vi "sv_UFF58 Check Channel Names.vi"(0 "abscissa channel name":string, 5 "ordinate numerator channel name":string, 7 "ordinate denominator channel name":string) -> (4 "abscissa channel name out":string, 6 "ordinate numerator channel name out":string, 8 "ordinate denominator channel name out":string)   [LabVIEW 2017, in "SoundVib_UFF58.lvlib"]
uses:
  <vilib>/addons/Sound and Vibration/svt_UFF58/SoundVib_UFF58.lvlib
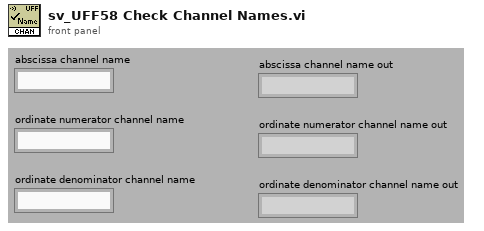
[diagram p1: front panel]
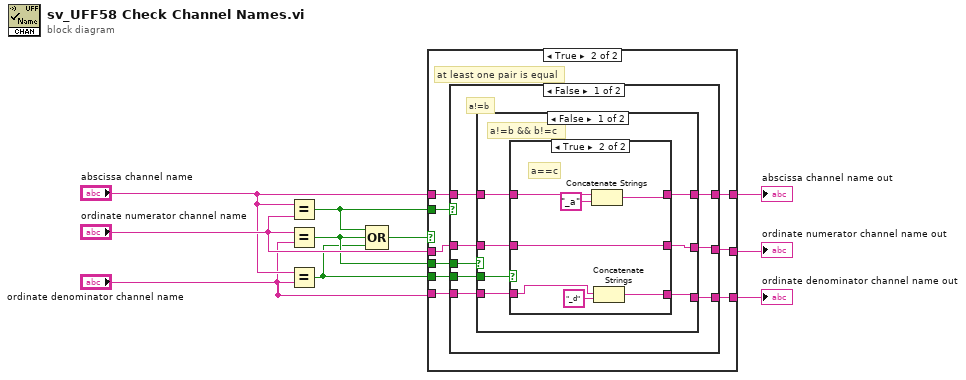
[diagram p0: block diagram]
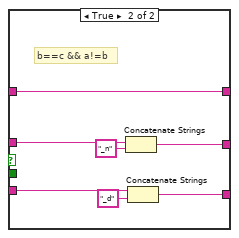
[diagram p4: hidden frame]
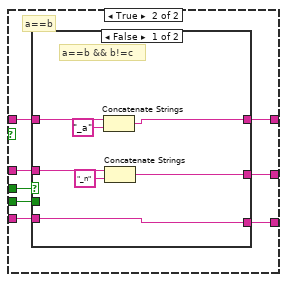
[diagram p5: hidden frame]
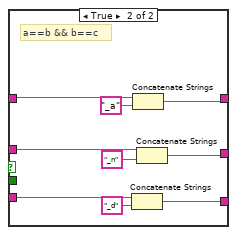
[diagram p6: hidden frame]
diagram:
  n1 = Equal?(x="abscissa channel name", y="ordinate numerator channel name") -> (x = y?=w6:bool)
  n2 = Equal?(x="ordinate numerator channel name", y="ordinate denominator channel name") -> (x = y?=w5:bool)
  n3 = Equal?(x="abscissa channel name", y="ordinate denominator channel name") -> (x = y?=w4:bool)
  n4 = Compound Arithmetic op=OR(w6, w5, w4) -> (w7:bool)
  n5 = case shown="True" w7 {
    tunnel: "ordinate numerator channel name" -> [w12 w18]
    tunnel: "ordinate denominator channel name" -> [w11 w16]
    tunnel: "abscissa channel name" -> [w13 w20]
    tunnel: w5 -> [_ w21]
    tunnel: w6 -> [_ w22]
    tunnel: [w13 w19] -> w3
    tunnel: [w12 w17] -> w2
    tunnel: [w11 w15] -> w1
    tunnel: w4 -> [_ w14]
    frame False {
      # "a!=b!=c"
    }
    frame True {
      # "at least one pair is equal"
      n6 = case shown="False" w22 {
        tunnel: w21 -> [w30 w62]
        tunnel: w20 -> [w25 w61]
        tunnel: [w24 w60] -> w19
        tunnel: w18 -> [w29 w59]
        tunnel: [w27 w58] -> w17
        tunnel: w16 -> [w28 w57]
        tunnel: [w26 w56] -> w15
        tunnel: w14 -> [w23 w55]
        frame False {
          # "a!=b"
          n7 = case shown="False" w30 {
            tunnel: w29 -> [w35 w52]
            tunnel: w28 -> [w34 w51]
            tunnel: [w32 w50] -> w27
            tunnel: [w31 w49] -> w26
            tunnel: w25 -> [w36 w48]
            tunnel: [w33 w48] -> w24
            tunnel: w23 -> [w37 _]
            frame False {
              # "a!=b && b!=c"
              n8 = case shown="True" w37 {
                tunnel: w36 -> [w40 w45]
                tunnel: w35 -> [w39 w43]
                tunnel: w34 -> [w38 w42]
                tunnel: [w40 w44] -> w33
                tunnel: [w39 w43] -> w32
                tunnel: [w38 w41] -> w31
                frame False {
                }
                frame True {
                  # "a==c"
                  n9 = Concatenate Strings(w45, "_a" ("string")) -> (w44:string)
                  n10 = Concatenate Strings(w42, "_d" ("string")) -> (w41:string)
                }
              }
            }
            frame True {
              # "b==c && a!=b"
              n11 = Concatenate Strings(w52, "_n" ("string")) -> (w50:string)
              n12 = Concatenate Strings(w51, "_d" ("string")) -> (w49:string)
            }
          }
        }
        frame True {
          # "a==b"
          n13 = case shown="False" w62 {
            tunnel: w61 -> [w69 w76]
            tunnel: [w67 w77] -> w60
            tunnel: w59 -> [w65 w75]
            tunnel: [w64 w74] -> w58
            tunnel: w57 -> [w63 w70]
            tunnel: [w63 w71] -> w56
            tunnel: w55 -> [_ _]
            frame False {
              # "a==b && b!=c"
              n14 = Concatenate Strings(w69, "_a" ("string")) -> (w67:string)
              n15 = Concatenate Strings(w65, "_n" ("string")) -> (w64:string)
            }
            frame True {
              # "a==b && b==c"
              n16 = Concatenate Strings(w70, "_d" ("string")) -> (w71:string)
              n17 = Concatenate Strings(w76, "_a" ("string")) -> (w77:string)
              n18 = Concatenate Strings(w75, "_n" ("string")) -> (w74:string)
            }
          }
        }
      }
    }
  }
  "ordinate numerator channel name out" <- w2
  "ordinate denominator channel name out" <- w1
  "abscissa channel name out" <- w3
